vi "Hindbrain.vi"() -> ()   [LabVIEW 2011]
uses:
  <vilib>/NXT/Subs/LVHSConnector.ctl
  <vilib>/NXT/Block Support/NXT_InputPort.ctl
  <vilib>/NXT/HiTechnic/HiTechnic Controls/HiTechnic Port.ctl
  <vilib>/NXT/Block Support/NXT_MessageMailbox.ctl
  <vilib>/NXT/Dual Mode Library/Waits/Wait_Num(msec).vi
  <vilib>/NXT/Dual Mode Library/Display/drawNumber.vi
  <vilib>/NXT/Dual Mode Library/Display/drawNumber_float.vi
  Hindbrain/mindsensors.com_LVEE_Toolkit_V1.23/mindsensors.com LVEE Toolkit/Dual/NXTServo-DM.vi
  <vilib>/NXT/HiTechnic/HiTechnic SubVIs/HiTechnic IRSeeker Sensor_DC_dir.vi
  Hindbrain/mindsensors.com_LVEE_Toolkit_V1.23/mindsensors.com LVEE Toolkit/Dual/NXTSumoEyes-DM.vi
  Hindbrain/mindsensors.com_LVEE_Toolkit_V1.23/mindsensors.com LVEE Toolkit/Dual/Distance Sensor-DM.vi
  <vilib>/NXT/Dual Mode Library/BT/BlueTooth_Write_String_toComputer.vi
panel:
  in  "NXT":T1={"Hardware"="NXT", "Flattened String"=""}
  out "IR Seeker":i16
  out "Distance Sensor":cluster{"Distance Value":ext, "Status":bool}
  out "Sumo Eyes":i16 caption="Scaled Value"
  out "Left?":bool
  out "Right?":bool
  out "Front?":bool
  out "Stuff?":bool
  in  "stop":bool
  in  "Propeller Servo":T2={"Servo Number"=1, "Position"=1500, "Speed"=0} {"Speed" step=1 scale=0.0..255.0; "Position" min=500 max=2500 step=1 scale=500.0..2500.0; "Servo Number" min=1 max=8 step=1}
  in  "Rudder Servo":T2={"Servo Number"=1, "Position"=1500, "Speed"=0} {"Speed" step=1 scale=0.0..255.0; "Position" min=500 max=2500 step=1 scale=500.0..2500.0; "Servo Number" min=1 max=8 step=1}
  out "Rudder Output":cluster{"Voltage":u8, "Status":bool}
  out "Propeller Output":cluster{"Voltage":u8, "Status":bool}
  # "Direction (0-9)"
  # "Scaled Value"
  # "Instructions:\n\nYou can run this Vi in two modes:\n\nA) Remote Mode (entirely embedded in NXT..you will need to run midbrain to get data)\n     i) Run NXT Terminal (under tools) and scan to see which NXT you're connected to\n     ii) Right click the box on the lower left hand corner of this VI and choose the \n         target you want to download the code onto\n     iii) Run the midbrain VI to communicate with the NXT\n\nB) Direct Mode (VI will run on this computer and communicate with NXT as an external\n     device)\n     i) Enter your NXT name under \"NXT\" box (green)\n     ii) Right now the motor is waiting for data sent by the midbrain.  You can rewire the \n         block diagram to connect the servo motor input to the Rudder Servo and Propeller\n         Servo controls\n     iii) You should be able t see the sensors feedback regardless"
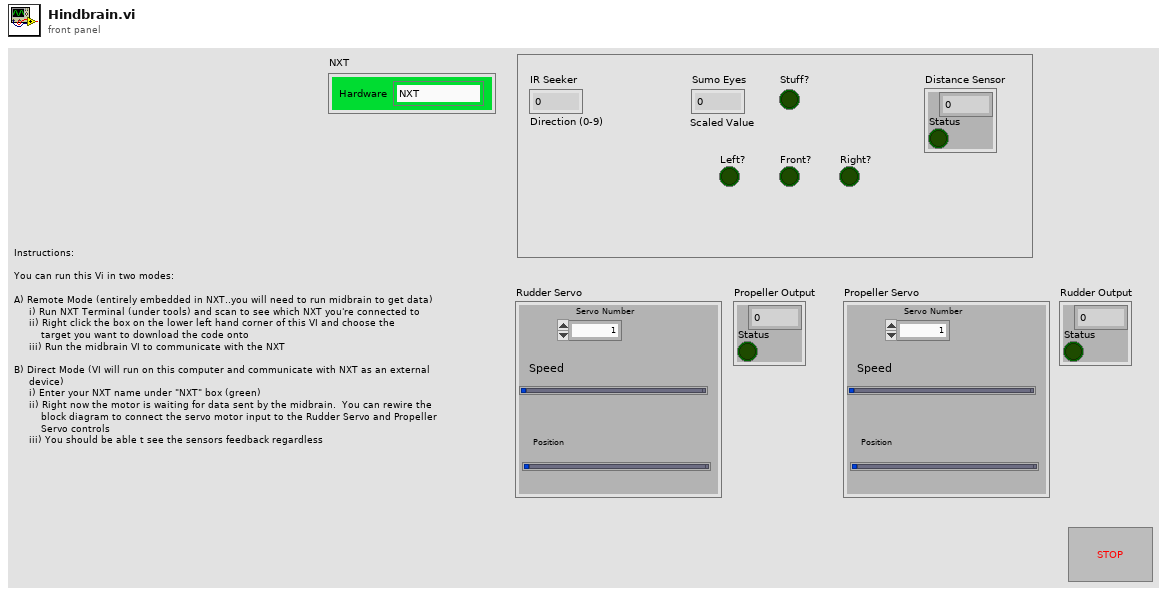
[diagram p1: front panel]
types:
  T1 = typedef "LVHSConnector.ctl" = cluster{"Hardware":string, "Flattened String":string}
  T2 = cluster{"Servo Number":u8, "Position":u16, "Speed":u8}
  T3 = typedef "HiTechnic Port.ctl" = cluster{"Port":T4, "MUX Port":u8}
  T4 = typedef "NXT_InputPort.ctl" = u8
  T5 = typedef "NXT_MessageMailbox.ctl" = u8
  T6 = cluster{"Which Zone?":u8, "Scaled Value":i16, "Status":bool}
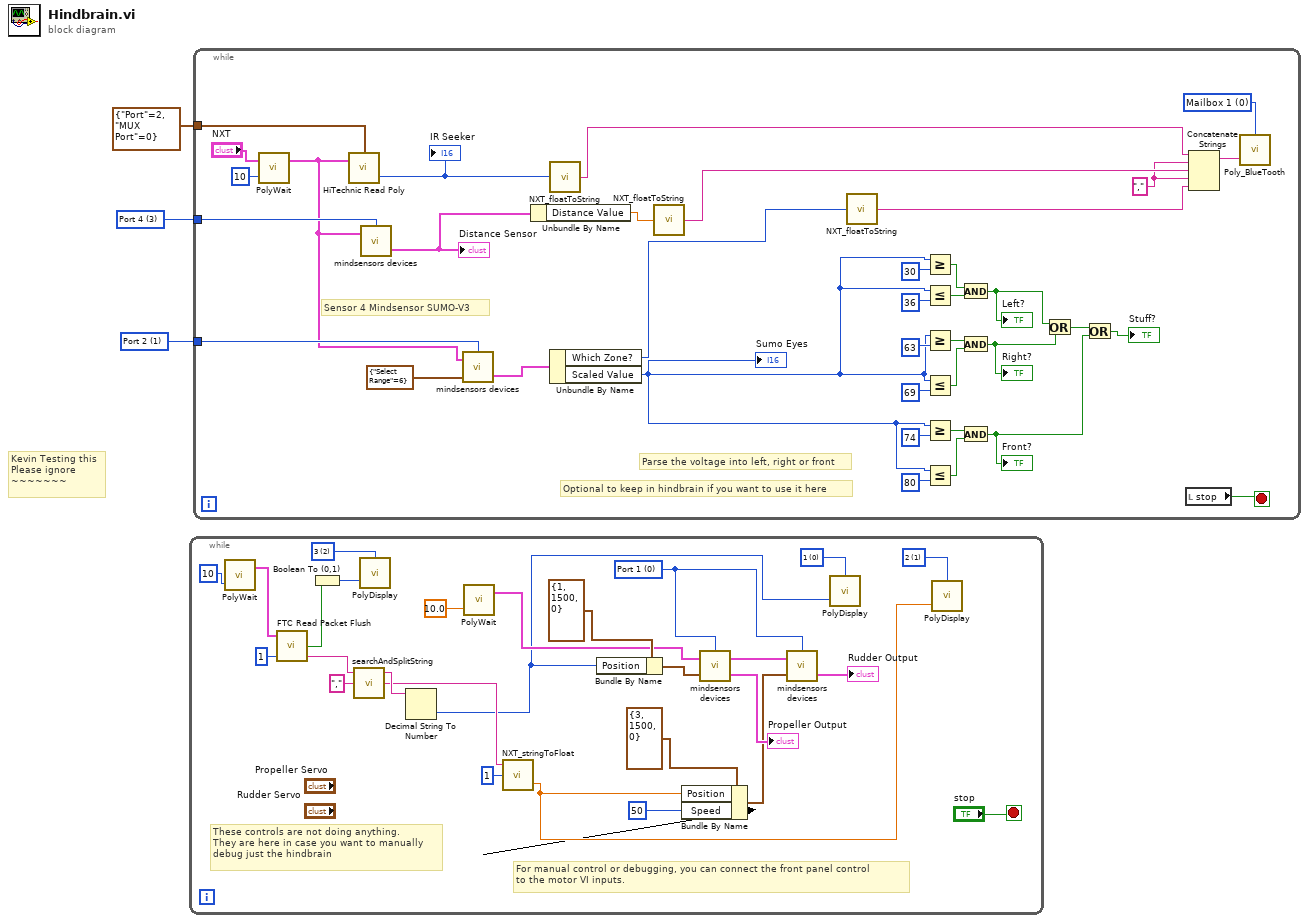
[diagram p0: block diagram]
diagram:
  w2 = T4 1 items=["Port 1", "Port 2", "Port 3", "Port 4"] ("Input Port")
  w3 = T4 3 items=["Port 1", "Port 2", "Port 3", "Port 4"] ("Input Port")
  # "Kevin Testing this\nPlease ignore\n~~~~~~~"
  n1 = while {
    stop <- "stop" stop-if-true
    w6 = i16 2 items=["1", "2", "3", "4", "5", "6", "7", "8"] ("Line")
    w11 = i16 1 items=["1", "2", "3", "4", "5", "6", "7", "8"] ("Line")
    w13 = i16 0 items=["1", "2", "3", "4", "5", "6", "7", "8"] ("Line")
    w23 = T4 0 items=["Port 1", "Port 2", "Port 3", "Port 4"] ("Input Port")
    # "These controls are not doing anything.\nThey are here in case you want to manually\ndebug just the hindbrain"
    # "For manual control or debugging, you can connect the front panel control\nto the motor VI inputs."
    n2 = call-poly <vilib>:"PolyWait.vi"("Time (100 msec)"=u32 10) -> ("NXT"=w9:T1)  [unwired: 3 in]
    n3 = call "FTC Read Packet Flush.vi"("Packet Length"=1, "NXT"=w9) -> ("Message"=w8:string, "Packet Received?"=w4:bool)  [unwired: 1 in, 1 out]
    n4 = Boolean To (0,1)(Boolean=w4) -> (0, 1=w5:i16)
    n5 = call <vilib>:"searchAndSplitString.vi"("search string/char (-)"=",", "string"=w8) -> ("match + rest of string"=w17:string, "substring before match"=w18:string)  [unwired: 1 in, 1 out]
    n6 = call-poly <vilib>:"PolyDisplay.vi"("number"=w5, "Line"=w6) -> ()  [unwired: 2 in, 1 out]
    n7 = Decimal String To Number(string=w18) -> (number=w14:i32)  [unwired: 2 in, 1 out]
    n8 = call-poly <vilib>:"PolyWait.vi"("Time (100 msec)"=sgl 10.0 ("Time (1 sec)")) -> ("NXT"=w20:T1)  [unwired: 3 in]
    n9 = call <vilib>:"NXT_stringToFloat.vi"("offset"=1, "string"=w17) -> ("number"=w12:sgl)  [unwired: 1 in, 1 out]
    n10 = Bundle By Name(cluster=T2 {"Servo Number"=1, "Position"=1500, "Speed"=0} ("Input of NXTServo"), "Position"=w14) -> (w27:T2)
    n11 = Bundle By Name(cluster=T2 {"Servo Number"=3, "Position"=1500, "Speed"=0} ("Input of NXTServo"), "Position"=w12, "Speed"=u8 50) -> (w24:T2)
    n12 = call-poly "mindsensors devices.vi"("Input of NXTServo"=w27, "NXT"=w20, "Input Port"=w23) -> ("Output of NXTServo"=→"Propeller Output":cluster{"Voltage":u8, "Status":bool}, "NXT dup"=w30:T1)
    n13 = call-poly "mindsensors devices.vi"("Input of NXTServo"=w24, "NXT"=w30, "Input Port"=w23) -> ("Output of NXTServo"=→"Rudder Output":cluster{"Voltage":u8, "Status":bool})  [unwired: 1 out]
    n14 = call-poly <vilib>:"PolyDisplay.vi"("number"=w14, "Line"=w13) -> ()  [unwired: 2 in, 1 out]
    n15 = call-poly <vilib>:"PolyDisplay.vi"("number"=w12, "Line"=w11) -> ()  [unwired: 2 in, 1 out]
  }
  n16 = while {
    tunnel: w3 -> [w66]
    tunnel: w2 -> [w49]
    tunnel: T3 {"Port"=2, "MUX Port"=0} ("Port/MUX") -> [w48]
    stop <- w67 stop-if-true
    w36 = T5 0 items=["Mailbox 1", "Mailbox 2", "Mailbox 3", "Mailbox 4", "Mailbox 5", "Mailbox 6", "Mailbox 7", "Mailbox 8", "Mailbox 9", "Mailbox 10"] ("Mailbox")
    w39 = "," ("string")
    # "Optional to keep in hindbrain if you want to use it here"
    # "Sensor 4 Mindsensor SUMO-V3"
    # "Parse the voltage into left, right or front"
    n17 = call-poly <vilib>:"PolyWait.vi"("Time (100 msec)"=u32 10, "NXT"="NXT") -> ("NXT"=w47:T1)  [unwired: 2 in]
    n18 = call-poly <vilib>:"HiTechnic Read Poly.vi"("NXT"=w47, "Port/MUX"=w48) -> ("Direction (0-9)"=w44:i16)  [unwired: 1 in, 1 out]
    "IR Seeker" <- w44
    n19 = call-poly "mindsensors devices.vi"("NXT"=w47, "Input Port"=w66) -> ("Output of Distance Sensor"=w45:cluster{"Distance Value":ext, "Status":bool})  [unwired: 1 in, 1 out]
    "Distance Sensor" <- w45
    n20 = call-poly "mindsensors devices.vi"("Input of NXTSumoEyes"=cluster{"Select Range":u16} {"Select Range"=6}, "NXT"=w47, "Input Port"=w49) -> ("Output of NXTSumoEyes"=w51:T6)  [unwired: 1 out]
    n21 = Unbundle By Name(w45) -> ("Distance Value"=w43:ext)
    n22 = call <vilib>:"NXT_floatToString.vi"("number"=w44) -> ("string"=w41:string)
    n23 = Unbundle By Name(w51) -> ("Which Zone?"=w31:u8, "Scaled Value"=w42:i16)
    "Sumo Eyes" <- w42
    n24 = call <vilib>:"NXT_floatToString.vi"("number"=w43) -> ("string"=w40:string)
    n25 = call <vilib>:"NXT_floatToString.vi"("number"=w31) -> ("string"=w38:string)
    n26 = Greater Or Equal?(x=w42, y=i16 30) -> (x >= y?=w63:bool)
    n27 = Less Or Equal?(x=w42, y=i16 36) -> (x <= y?=w62:bool)
    n28 = Greater Or Equal?(x=w42, y=i16 63) -> (x >= y?=w60:bool)
    n29 = Less Or Equal?(x=w42, y=i16 69) -> (x <= y?=w61:bool)
    n30 = Greater Or Equal?(x=w42, y=i16 74) -> (x >= y?=w56:bool)
    n31 = Less Or Equal?(x=w42, y=i16 80) -> (x <= y?=w57:bool)
    n32 = And(x=w63, y=w62) -> (x .and. y?=w34:bool)
    "Left?" <- w34
    n33 = And(x=w60, y=w61) -> (x .and. y?=w32:bool)
    "Right?" <- w32
    n34 = And(x=w56, y=w57) -> (x .and. y?=w33:bool)
    "Front?" <- w33
    n35 = Or(x=w34, y=w32) -> (x .or. y?=w53:bool)
    n36 = Or(x=w53, y=w33) -> (x .or. y?=→"Stuff?":bool)
    n37 = local read "stop"() -> (w67:bool)
    n38 = Concatenate Strings(w41, w39, w40, w39, w38) -> (w37:string)
    n39 = call-poly <vilib>:"Poly_BlueTooth.vi"("Message in"=w37, "Mailbox"=w36) -> ()  [unwired: 2 in, 1 out]
  }
